vi "Process Value Delays.vi"(8 "Values":dbl[](array[numeric]), 9 "Delay":dbl, 10 "Time in Step":dbl, 11 "Mode":string) -> (3 "Value out":dbl)   [LabVIEW 2020, in "Output Sequencer.lvlib" / "Output Sequencer.lvclass"]
uses:
  Output Sequencer.lvclass
  Globals/Global Strings.vi
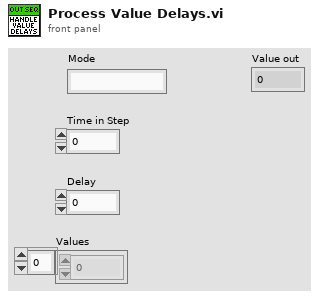
[diagram p1: front panel]
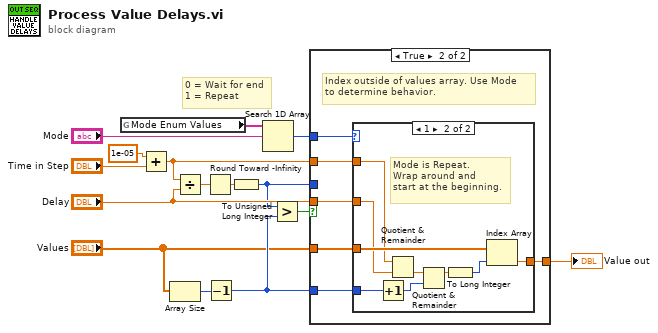
[diagram p0: block diagram]
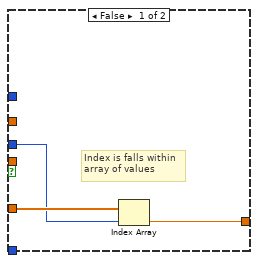
[diagram p2: hidden frame]
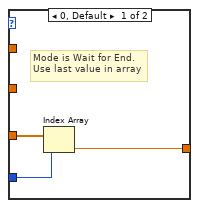
[diagram p3: hidden frame]
diagram:
  # "0 = Wait for end\n1 = Repeat"
  n1 = global read "Global Strings.vi" "Mode Enum Values"() -> (w3:string[])
  n2 = Add(x=1e-05, y="Time in Step") -> (x+y=w15:dbl)
  n3 = Array Size(array="Values") -> (size(s)=w4:i32)
  n4 = Divide(x=w15, y="Delay") -> (x/y=w12:dbl)
  n5 = Round Toward -Infinity(1:w12) -> (0:w7:dbl)
  n6 = Decrement(x=w4) -> (x-1=w10:i32)
  n7 = To Unsigned Long Integer(number=w7) -> (unsigned 32bit integer=w8:u32)
  n8 = Search 1D Array(1D array=w3, element="Mode") -> (index of element=w2:i32)  [unwired: 1 in]
  n9 = Greater?(x=w8, y=w10) -> (0:w6:bool)
  n10 = case shown="True" w6 {
    tunnel: "Values" -> [w18 w23]
    tunnel: w8 -> [w17 _]
    tunnel: [w16 w21] -> w9
    tunnel: w2 -> [_ w24]
    tunnel: w10 -> [_ w22]
    tunnel: "Delay" -> [_ w20]
    tunnel: w15 -> [_ w19]
    frame False {
      # "Index is falls within\narray of values"
      n11 = Index Array(array=w18, index=w17) -> (element=w16:dbl)
    }
    frame True {
      # "Index outside of values array. Use Mode\nto determine behavior."
      n12 = case shown="1" w24 {
        tunnel: w23 -> [w27 w36]
        tunnel: w22 -> [w26 w33]
        tunnel: [w25 w35] -> w21
        tunnel: w20 -> [_ w29]
        tunnel: w19 -> [_ w28]
        frame 0, Default {
          # "Mode is Wait for End.\nUse last value in array"
          n13 = Index Array(array=w27, index=w26) -> (element=w25:dbl)
        }
        frame 1 {
          # "Mode is Repeat.\nWrap around and \nstart at the beginning."
          n14 = Increment(x=w33) -> (x+1=w32:i32)
          n15 = Quotient & Remainder(x=w28, y=w29) -> (floor(x/y)=w34:dbl)  [unwired: 1 out]
          n16 = Quotient & Remainder(x=w34, y=w32) -> (x-y*floor(x/y)=w31:dbl)  [unwired: 1 out]
          n17 = To Long Integer(number=w31) -> (32bit integer=w30:i32)
          n18 = Index Array(array=w36, index=w30) -> (element=w35:dbl)
        }
      }
    }
  }
  "Value out" <- w9
